vi "Config Type.vi"(11 "Command in":refnum<class "Command.lvclass">) -> (2 "Command Config Type":refnum<class "Command Config.lvclass">)   [LabVIEW 2020, in "VolatusSeq.lvlib" / "Command.lvclass"]
uses:
  Command.lvclass
  Command.lvclass/Command.ctl
  VolatusSeqConfig/Command Config/Command Config.lvclass
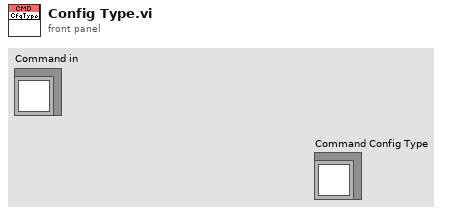
[diagram p1: front panel]
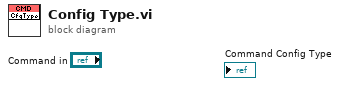
[diagram p0: block diagram]
diagram:
